vi "Write Scope.vi"(8 "error in (no error)":errorcluster, 10 "Scope":variant, 11 "Callback in":refnum<class "Callback.lvclass">) -> (0 "error out":errorcluster, 3 "Callback out":refnum<class "Callback.lvclass">)   [LabVIEW 2017, in "Promise Future.lvlib" / "Callback.lvclass"]
uses:
  Callback.lvclass
  Callback.lvclass/Callback.ctl
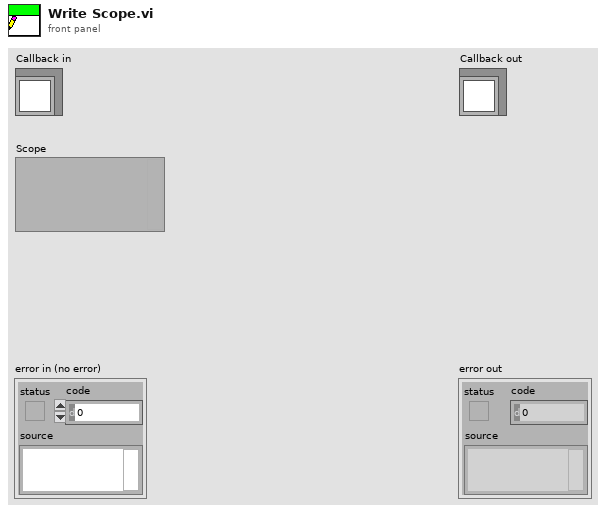
[diagram p1: front panel]
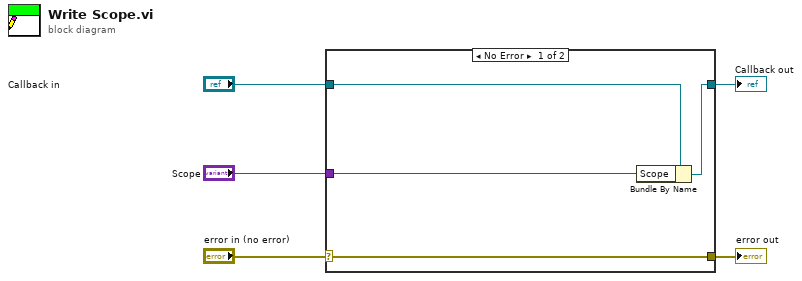
[diagram p0: block diagram]
diagram:
  n1 = case shown="No Error" "error in (no error)" {
    selector: "error in (no error)" -> [w9 w10]
    tunnel: [w9 w10] -> w4
    tunnel: [w7 w11] -> w2
    tunnel: "Callback in" -> [w8 w11]
    tunnel: "Scope" -> [w6 _]
    frame No Error {
      n2 = Bundle By Name(cluster=w8, "Scope"=w6) -> (w7:refnum<class "Callback.lvclass">)
    }
    frame Error {
    }
  }
  "error out" <- w4
  "Callback out" <- w2
